vi "Shooting.vi"(11 "input cluster":T2) -> (3 "Shooter Info Cluster":T1)   [LabVIEW 2015]
uses:
  Joystick/ControlsToCommands.ctl
  References/Refnums.vi
panel:
  in  "Shooter Info":T1
  in  "Time Indexing before Turning off Motors":dbl=3.0 caption="Delay Time (s)"
  in  "Time Spinning before Index":dbl=5.0 caption="Delay Time (s)"
  in  "Shooting":u16(ring) items=["Normal Operation", "Autonomous Shooting"]
  in  "Motor Power":dbl min=-1.0 max=1.0 step=1.0
  # "For Autonomous Shooting"
  # "For Normal Operation"
  # "WARNING THIS SHOOT FUNCTION CANNOT BE ABORTED\nIT WILL FOLLOW THROUGH UNTIL IT IS FINISHED"
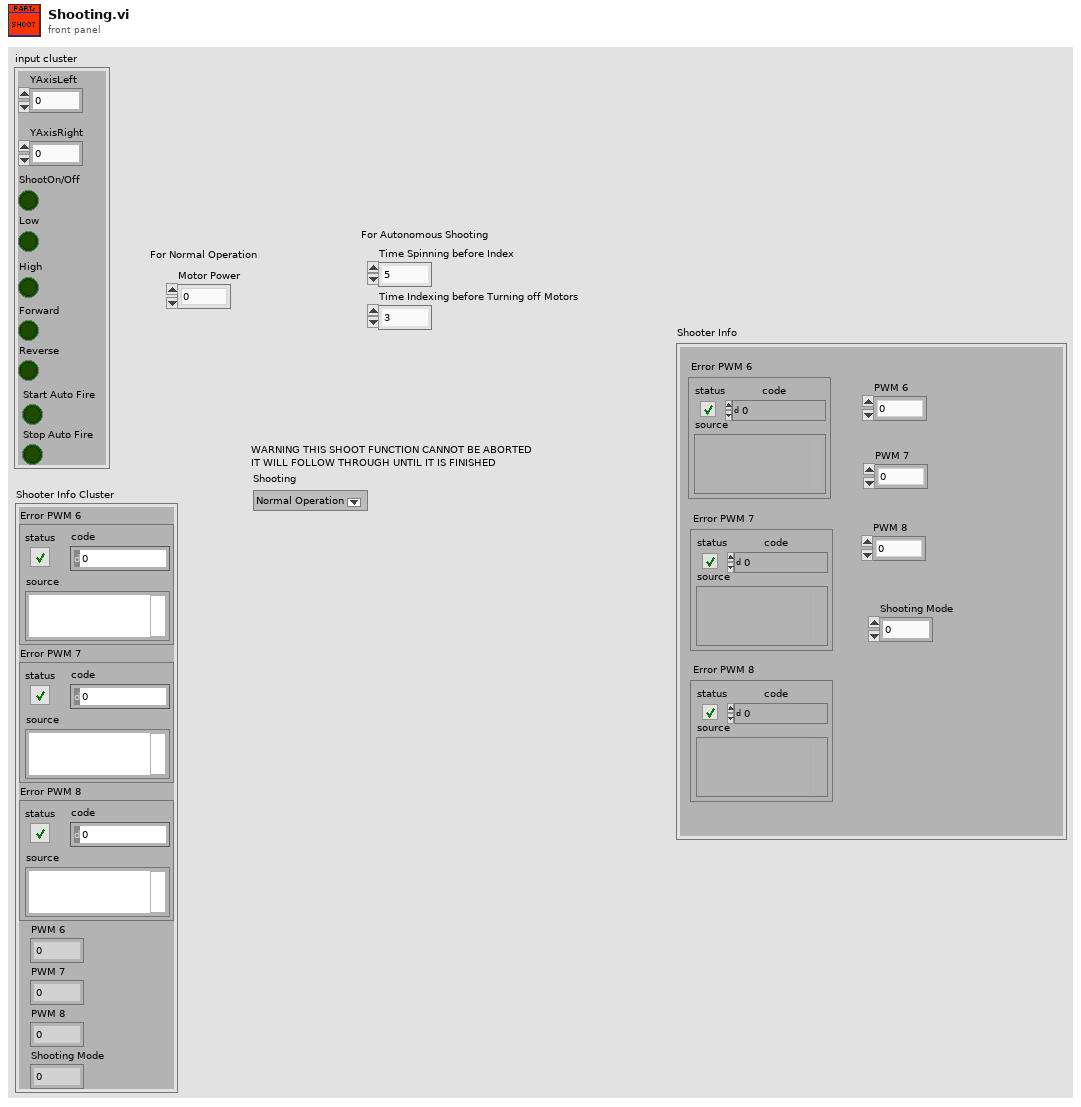
[diagram p1: front panel]
types:
  T1 = cluster{"Error PWM 6":errorcluster, "Error PWM 7":errorcluster, "Error PWM 8":errorcluster, "PWM 6":dbl, "PWM 7":dbl, "PWM 8":dbl, "Shooting Mode":dbl}
  T2 = typedef "ControlsToCommands.ctl" = cluster{"YAxisLeft":dbl, "YAxisRight":dbl, "ShootOn/Off":bool, "Low":bool, "High":bool, "Forward":bool, "Reverse":bool, "Start Auto Fire":bool, "Stop Auto Fire":bool}
  T3 = typedef "WPI_MotorControlDeviceRef.ctl" = cluster{"DeviceStatus":errorcluster, "Type":T4, "PWM":cluster{"PWM Channel":T5, "DeadBand":T6}, "CAN":cluster{"Device Number":u8, "Control Mode":T7, "Semaphore":T8, "Max Vout":dbl, "TalonSRX Control Mode":T9}, "Invert":bool}
  T4 = typedef "WPI_MotorControlType.ctl" = enum16{"PWM", "CAN", "CANTalonSRX"}
  T5 = typedef "FPGA_DIOPWMChannel.ctl" = enum8{"PWM 0", "PWM 1", "PWM 2", "PWM 3", "PWM 4", "PWM 5", "PWM 6", "PWM 7", "PWM 8", "PWM 9", "PWM MXP 0", "PWM MXP 1", "PWM MXP 2", "PWM MXP 3", "PWM MXP 4", "PWM MXP 5", "PWM MXP 6", "PWM MXP 7", "PWM MXP 8", "PWM MXP 9", "Invalid"}
  T6 = typedef "WPI_PWMDeadband.ctl" = cluster{"Name":string, "maxPositivePwm":i32, "minPositivePwm":i32, "centerPwm":i32, "maxNegativePwm":i32, "minNegativePwm":i32, "angularRange":u16}
  T7 = typedef "WPI_CANJaguar_ControlMode.ctl" = enum8{"Percent VBus", "Current", "Speed", "Position", "Voltage"}
  T8 = typedef "Semaphore RefNum" = refnum<k1>
  T9 = typedef "WPI_CANTalonSRX_APIControlMode.ctl" = enum8{"Percent VBus", "Speed", "Position", "Slave", "Unchanged / Invalid", "Voltage Compensation", "Current", "Motion Profile"}
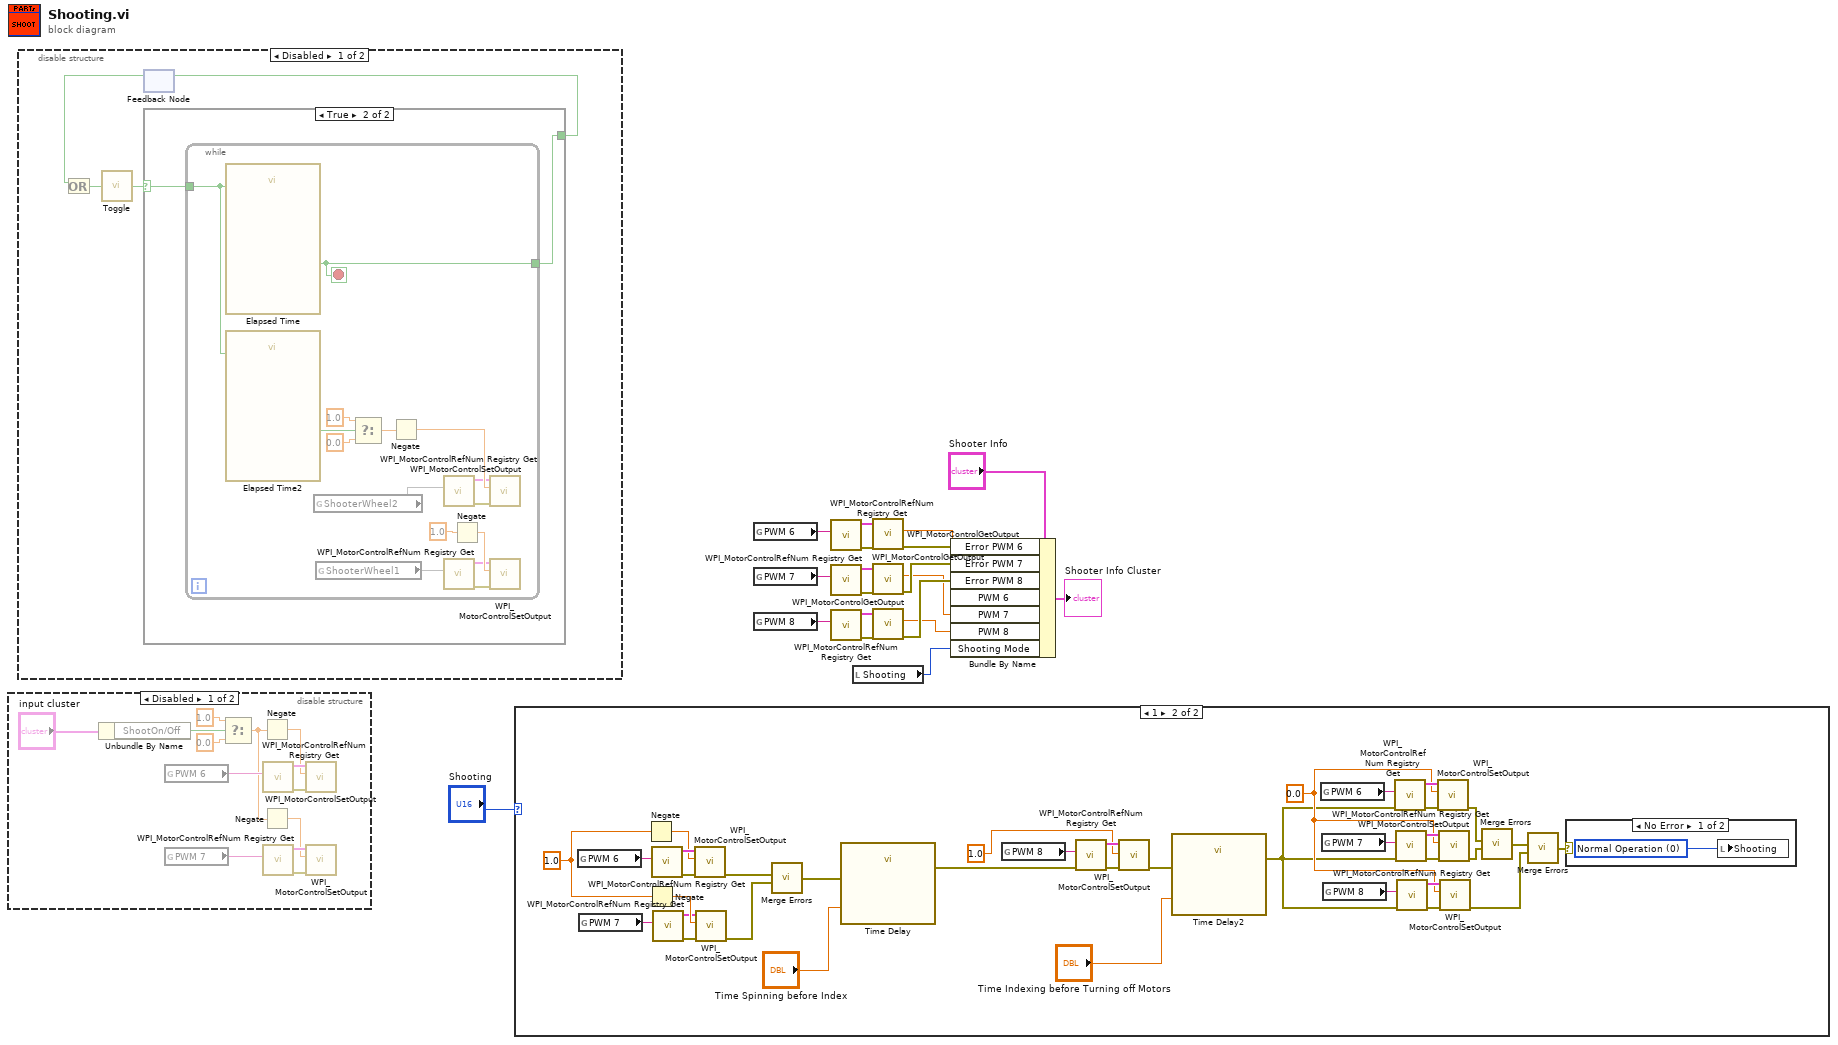
[diagram p0: block diagram]
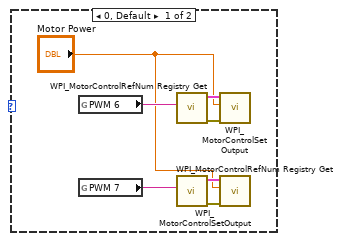
[diagram p2: hidden frame]
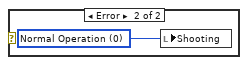
[diagram p3: hidden frame]
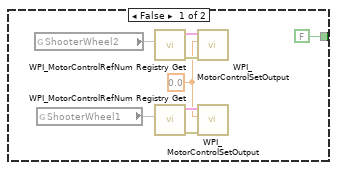
[diagram p5: hidden frame]
diagram:
  n1 = disable-structure shown="Disabled" {
    frame Disabled {
      n2 = Unbundle By Name("input cluster") -> ("ShootOn/Off"=w22:bool)
      n3 = global read "Refnums.vi" "PWM 6"() -> (w28:string)
      n4 = global read "Refnums.vi" "PWM 7"() -> (w29:string)
      n5 = Select(t=1.0, s=w22, f=0.0) -> (s? t:f=w20:dbl)
      n6 = Negate(x=w20) -> (-x=w21:dbl)
      n7 = Negate(x=w20) -> (-x=w25:dbl)
      n8 = call <vilib>:"WPI_MotorControlRefNum Registry Get.vi"("refnum name"=w28) -> ("error out"=w27:errorcluster, "MotorControlDevRef"=w26:T3)  [unwired: 9 in]
      n9 = call <vilib>:"WPI_MotorControlRefNum Registry Get.vi"("refnum name"=w29) -> ("error out"=w31:errorcluster, "MotorControlDevRef"=w30:T3)  [unwired: 9 in]
      n10 = call <vilib>:"WPI_MotorControlSetOutput.vi"("error in (no error)"=w27, "Output"=w21, "MotorControlDevRef"=w26) -> ()  [unwired: 6 in, 3 out]
      n11 = call <vilib>:"WPI_MotorControlSetOutput.vi"("error in (no error)"=w31, "Output"=w25, "MotorControlDevRef"=w30) -> ()  [unwired: 6 in, 3 out]
    }
    frame Enabled {
    }
  }
  n12 = disable-structure shown="Disabled" {
    frame Disabled {
      n13 = feedback #1() -> (w33:bool)  [unwired: 1 in]
      n14 = Or(x=w33) -> (x .or. y?=w36:bool)  [unwired: 1 in]
      n15 = call "Toggle.vi"("Input"=w36) -> ("Output"=w35:bool)  [unwired: 4 in]
      n16 = case shown="True" w35 {
        selector: w35 -> [_ w46]
        tunnel: [FALSE ("Time has Elapsed") w45] -> w34
        frame False {
          w38 = 0.0 ("Output")
          n17 = global read "Refnums.vi" "ShooterWheel2"() -> (w42)
          n18 = global read "Refnums.vi" "ShooterWheel1"() -> (w41)
          n19 = call <vilib>:"WPI_MotorControlRefNum Registry Get.vi"("refnum name"=w42) -> ("error out"=w44:errorcluster, "MotorControlDevRef"=w43:T3)  [unwired: 9 in]
          n20 = call <vilib>:"WPI_MotorControlRefNum Registry Get.vi"("refnum name"=w41) -> ("error out"=w39:errorcluster, "MotorControlDevRef"=w40:T3)  [unwired: 9 in]
          n21 = call <vilib>:"WPI_MotorControlSetOutput.vi"("error in (no error)"=w44, "Output"=w38, "MotorControlDevRef"=w43) -> ()  [unwired: 6 in, 3 out]
          n22 = call <vilib>:"WPI_MotorControlSetOutput.vi"("error in (no error)"=w39, "Output"=w38, "MotorControlDevRef"=w40) -> ()  [unwired: 6 in, 3 out]
        }
        frame True {
          n23 = while {
            tunnel: w46 -> [w48]
            tunnel: [w47] -> w45
            stop <- w47 stop-if-true
            n24 = call "Elapsed Time"("Reset"=w48) -> ("Time has Elapsed"=w47:bool)  [unwired: 11 in, 7 out]
            n25 = call "Elapsed Time2"("Reset"=w48) -> ("Time has Elapsed"=w49:bool)  [unwired: 11 in, 7 out]
            n26 = global read "Refnums.vi" "ShooterWheel2"() -> (w57)
            n27 = global read "Refnums.vi" "ShooterWheel1"() -> (w56)
            n28 = Select(t=1.0, s=w49, f=0.0) -> (s? t:f=w52:dbl)
            n29 = Negate(x=w52) -> (-x=w61:dbl)
            n30 = call <vilib>:"WPI_MotorControlRefNum Registry Get.vi"("refnum name"=w57) -> ("error out"=w59:errorcluster, "MotorControlDevRef"=w58:T3)  [unwired: 9 in]
            n31 = call <vilib>:"WPI_MotorControlRefNum Registry Get.vi"("refnum name"=w56) -> ("error out"=w54:errorcluster, "MotorControlDevRef"=w55:T3)  [unwired: 9 in]
            n32 = Negate(x=1.0) -> (-x=w60:dbl)
            n33 = call <vilib>:"WPI_MotorControlSetOutput.vi"("error in (no error)"=w59, "Output"=w61, "MotorControlDevRef"=w58) -> ()  [unwired: 6 in, 3 out]
            n34 = call <vilib>:"WPI_MotorControlSetOutput.vi"("error in (no error)"=w54, "Output"=w60, "MotorControlDevRef"=w55) -> ()  [unwired: 6 in, 3 out]
          }
        }
      }
      n35 = feedback-in #1(w34) -> ()
    }
    frame Enabled {
    }
  }
  n36 = case shown="1" "Shooting" {
    frame 0, Default {
      n37 = global read "Refnums.vi" "PWM 6"() -> (w66:string)
      n38 = global read "Refnums.vi" "PWM 7"() -> (w65:string)
      n39 = call <vilib>:"WPI_MotorControlRefNum Registry Get.vi"("refnum name"=w66) -> ("error out"=w67:errorcluster, "MotorControlDevRef"=w68:T3)  [unwired: 9 in]
      n40 = call <vilib>:"WPI_MotorControlRefNum Registry Get.vi"("refnum name"=w65) -> ("error out"=w63:errorcluster, "MotorControlDevRef"=w64:T3)  [unwired: 9 in]
      n41 = call <vilib>:"WPI_MotorControlSetOutput.vi"("error in (no error)"=w67, "Output"="Motor Power", "MotorControlDevRef"=w68) -> ()  [unwired: 6 in, 3 out]
      n42 = call <vilib>:"WPI_MotorControlSetOutput.vi"("error in (no error)"=w63, "Output"="Motor Power", "MotorControlDevRef"=w64) -> ()  [unwired: 6 in, 3 out]
    }
    frame 1 {
      w77 = 0.0
      w96 = 1.0
      n43 = global read "Refnums.vi" "PWM 6"() -> (w101:string)
      n44 = global read "Refnums.vi" "PWM 7"() -> (w100:string)
      n45 = Negate(x=w96) -> (-x=w97:dbl)
      n46 = Negate(x=w96) -> (-x=w104:dbl)
      n47 = call <vilib>:"WPI_MotorControlRefNum Registry Get.vi"("refnum name"=w101) -> ("error out"=w102:errorcluster, "MotorControlDevRef"=w103:T3)  [unwired: 9 in]
      n48 = call <vilib>:"WPI_MotorControlRefNum Registry Get.vi"("refnum name"=w100) -> ("error out"=w98:errorcluster, "MotorControlDevRef"=w99:T3)  [unwired: 9 in]
      n49 = call <vilib>:"WPI_MotorControlSetOutput.vi"("error in (no error)"=w102, "Output"=w97, "MotorControlDevRef"=w103) -> ("error out"=w95:errorcluster)  [unwired: 6 in, 2 out]
      n50 = call <vilib>:"WPI_MotorControlSetOutput.vi"("error in (no error)"=w98, "Output"=w104, "MotorControlDevRef"=w99) -> ("error out"=w94:errorcluster)  [unwired: 6 in, 2 out]
      n51 = call "Merge Errors.vi"("error in 2"=w94, "error in"=w95) -> ("error out"=w93:errorcluster)  [unwired: 2 in]
      n52 = call "Time Delay"("error in (no error)"=w93, "Delay Time (s)"="Time Spinning before Index") -> ("error out"=w89:errorcluster)  [unwired: 9 in]
      n53 = global read "Refnums.vi" "PWM 8"() -> (w92:string)
      n54 = call <vilib>:"WPI_MotorControlRefNum Registry Get.vi"("error in (no error)"=w89, "refnum name"=w92) -> ("error out"=w91:errorcluster, "MotorControlDevRef"=w90:T3)  [unwired: 8 in]
      n55 = call <vilib>:"WPI_MotorControlSetOutput.vi"("error in (no error)"=w91, "Output"=1.0, "MotorControlDevRef"=w90) -> ("error out"=w87:errorcluster)  [unwired: 6 in, 2 out]
      n56 = call "Time Delay2"("error in (no error)"=w87, "Delay Time (s)"="Time Indexing before Turning off Motors") -> ("error out"=w76:errorcluster)  [unwired: 9 in]
      n57 = global read "Refnums.vi" "PWM 6"() -> (w83:string)
      n58 = global read "Refnums.vi" "PWM 7"() -> (w84:string)
      n59 = global read "Refnums.vi" "PWM 8"() -> (w80:string)
      n60 = call <vilib>:"WPI_MotorControlRefNum Registry Get.vi"("error in (no error)"=w76, "refnum name"=w83) -> ("error out"=w82:errorcluster, "MotorControlDevRef"=w81:T3)  [unwired: 8 in]
      n61 = call <vilib>:"WPI_MotorControlRefNum Registry Get.vi"("error in (no error)"=w76, "refnum name"=w84) -> ("error out"=w86:errorcluster, "MotorControlDevRef"=w85:T3)  [unwired: 8 in]
      n62 = call <vilib>:"WPI_MotorControlRefNum Registry Get.vi"("error in (no error)"=w76, "refnum name"=w80) -> ("error out"=w78:errorcluster, "MotorControlDevRef"=w79:T3)  [unwired: 8 in]
      n63 = call <vilib>:"WPI_MotorControlSetOutput.vi"("error in (no error)"=w82, "Output"=w77, "MotorControlDevRef"=w81) -> ("error out"=w71:errorcluster)  [unwired: 6 in, 2 out]
      n64 = call <vilib>:"WPI_MotorControlSetOutput.vi"("error in (no error)"=w86, "Output"=w77, "MotorControlDevRef"=w85) -> ("error out"=w70:errorcluster)  [unwired: 6 in, 2 out]
      n65 = call <vilib>:"WPI_MotorControlSetOutput.vi"("error in (no error)"=w78, "Output"=w77, "MotorControlDevRef"=w79) -> ("error out"=w72:errorcluster)  [unwired: 6 in, 2 out]
      n66 = call "Merge Errors.vi"("error in 2"=w70, "error in"=w71) -> ("error out"=w73:errorcluster)  [unwired: 2 in]
      n67 = call "Merge Errors.vi"("error in 2"=w72, "error in"=w73) -> ("error out"=w69:errorcluster)  [unwired: 2 in]
      n68 = case shown="No Error" w69 {
        frame No Error {
          w105 = u16 0 items=["Normal Operation", "Autonomous Shooting"] ("Shooting")
          n69 = local write "Shooting"(w105) -> ()
        }
        frame Error {
          w106 = u16 0 items=["Normal Operation", "Autonomous Shooting"] ("Shooting")
          n70 = local write "Shooting"(w106) -> ()
        }
      }
    }
  }
  n71 = global read "Refnums.vi" "PWM 6"() -> (w18:string)
  n72 = global read "Refnums.vi" "PWM 7"() -> (w13:string)
  n73 = global read "Refnums.vi" "PWM 8"() -> (w12:string)
  n74 = call <vilib>:"WPI_MotorControlRefNum Registry Get.vi"("refnum name"=w18) -> ("error out"=w16:errorcluster, "MotorControlDevRef"=w17:T3)  [unwired: 9 in]
  n75 = call <vilib>:"WPI_MotorControlRefNum Registry Get.vi"("refnum name"=w13) -> ("error out"=w15:errorcluster, "MotorControlDevRef"=w14:T3)  [unwired: 9 in]
  n76 = call <vilib>:"WPI_MotorControlRefNum Registry Get.vi"("refnum name"=w12) -> ("error out"=w10:errorcluster, "MotorControlDevRef"=w11:T3)  [unwired: 9 in]
  n77 = local read "Shooting"() -> (w2:u16)
  n78 = call <vilib>:"WPI_MotorControlGetOutput.vi"("error in (no error)"=w16, "MotorControlDevRef"=w17) -> ("error out"=w8:errorcluster, "Output"=w5:dbl)  [unwired: 7 in, 1 out]
  n79 = call <vilib>:"WPI_MotorControlGetOutput.vi"("error in (no error)"=w15, "MotorControlDevRef"=w14) -> ("error out"=w7:errorcluster, "Output"=w4:dbl)  [unwired: 7 in, 1 out]
  n80 = call <vilib>:"WPI_MotorControlGetOutput.vi"("error in (no error)"=w10, "MotorControlDevRef"=w11) -> ("error out"=w6:errorcluster, "Output"=w3:dbl)  [unwired: 7 in, 1 out]
  n81 = Bundle By Name(cluster="Shooter Info", "Error PWM 6"=w8, "Error PWM 7"=w7, "Error PWM 8"=w6, "PWM 6"=w5, "PWM 7"=w4, "PWM 8"=w3, "Shooting Mode"=w2) -> (→"Shooter Info Cluster":T1)
